vi "TUNA midbrain THINK.vi"(3 "error in":errorcluster, 4 "Forebrain Comd":T2, 5 "IR Sensors":T3(array[cluster]), 6 "Camera Data":T1(array[cluster])) -> (0 "error out":errorcluster, 1 "Behavior\nVelocity OUT":dbl, 2 "Behavior arrays":T4)   [LabVIEW 2014]
doc: "This vi is the midbrain THINK routine. It selects the behaviors which the boat will use based upon the passed Forebrain Command."
panel:
  out "Waveform Graph":cluster{dbl, dbl, dbl[][]}(graph)
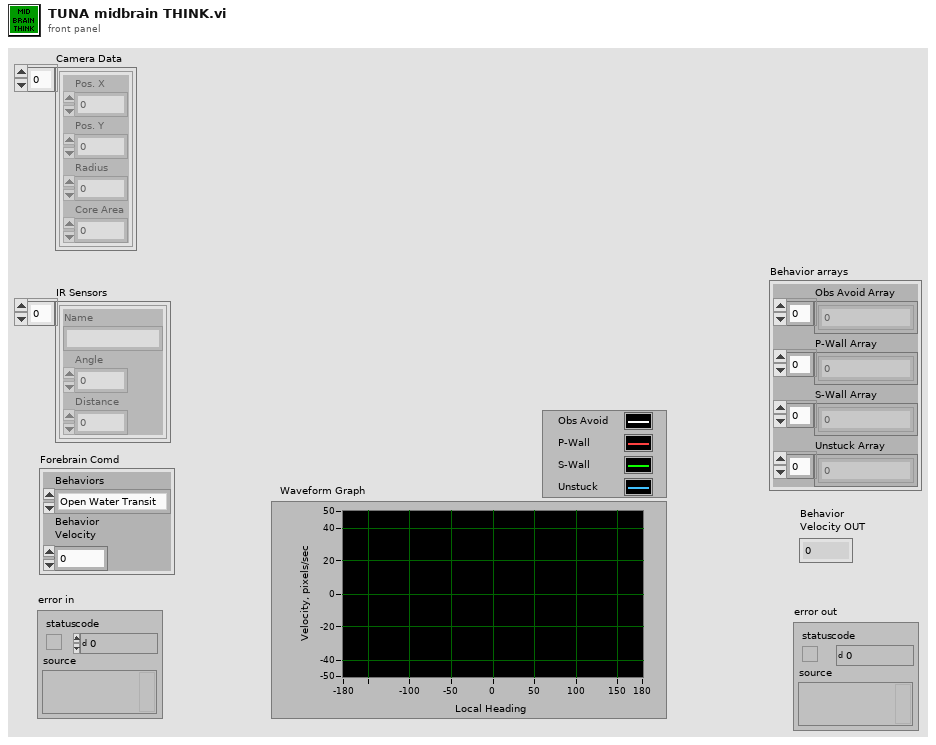
[diagram p1: front panel]
types:
  T1 = cluster{"Pos. X":i32, "Pos. Y":i32, "Radius":i32, "Core Area":i32}[]
  T2 = cluster{"Behaviors":enum16{"Open Water Transit", "P-Wall Follow", "S-Wall Follow", "Dock"}, "Behavior\nVelocity":dbl}
  T3 = cluster{"Name":string, "Angle":dbl, "Distance":dbl}[]
  T4 = cluster{"Obs Avoid Array":dbl[], "P-Wall Array":dbl[], "S-Wall Array":dbl[], "Unstuck Array":dbl[]}
  T5 = enum16{"Open Water Transit", "P-Wall Follow", "S-Wall Follow", "Dock"}
  T6 = cluster{"Obstacle Avoidance":bool, "P-Wall Follow":bool, "S-Wall Follow":bool, "Point to Dock":bool}
  T7 = cluster{"Obs Avoid Array":dbl[], "P-Wall Array":dbl[], "S-Wall Array":dbl[], "Dock Array":dbl[]}
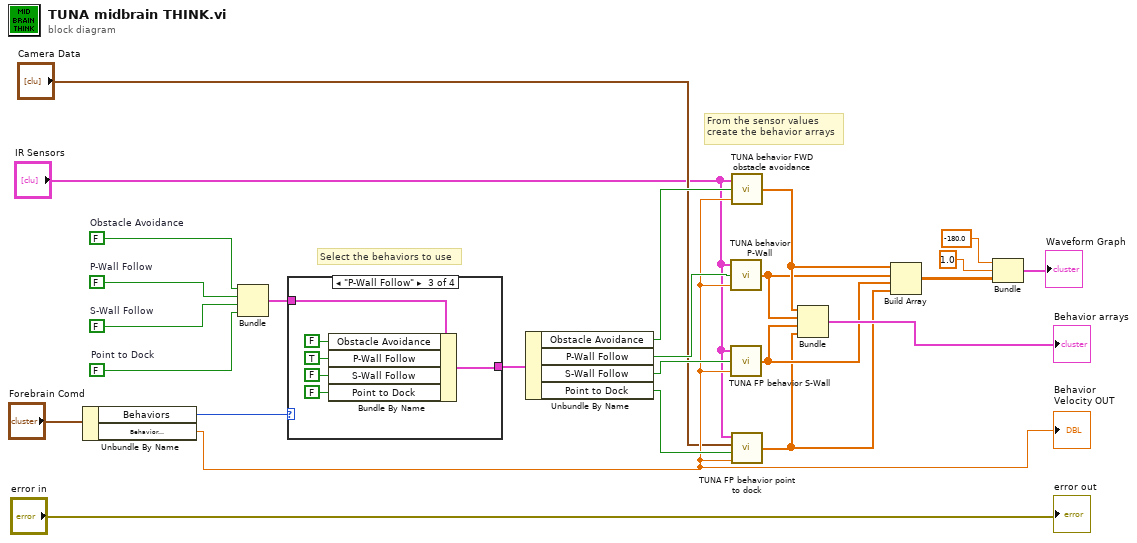
[diagram p0: block diagram]
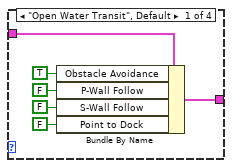
[diagram p2: hidden frame]
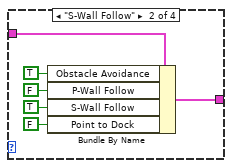
[diagram p3: hidden frame]
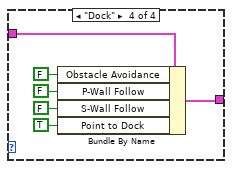
[diagram p4: hidden frame]
diagram:
  w21 = FALSE  # Point to Dock
  w22 = FALSE  # S-Wall Follow
  w23 = FALSE  # P-Wall Follow
  w24 = FALSE  # Obstacle Avoidance
  # "From the sensor values\ncreate the behavior arrays"
  # "Select the behaviors to use"
  n1 = Unbundle By Name("Forebrain Comd") -> ("Behaviors"=w4:T5, "Behavior\nVelocity"=w13:dbl)
  "Behavior\nVelocity OUT" <- w13
  n2 = Bundle("Obstacle Avoidance"=w24, "P-Wall Follow"=w23, "S-Wall Follow"=w22, "Point to Dock"=w21) -> (w20:T6)  [unwired: 1 in]
  n3 = case shown="\"P-Wall Follow\"" w4 {
    tunnel: w20 -> [w31 w37 w43 w49]
    tunnel: [w29 w35 w41 w47] -> w19
    frame "Open Water Transit", Default {
      n4 = Bundle By Name(cluster=w31, "Obstacle Avoidance"=TRUE, "P-Wall Follow"=FALSE, "S-Wall Follow"=FALSE, "Point to Dock"=FALSE ("Get Unstuck")) -> (w29:T6)
    }
    frame "S-Wall Follow" {
      n5 = Bundle By Name(cluster=w37, "Obstacle Avoidance"=TRUE, "P-Wall Follow"=FALSE, "S-Wall Follow"=TRUE, "Point to Dock"=FALSE ("Get Unstuck")) -> (w35:T6)
    }
    frame "P-Wall Follow" {
      n6 = Bundle By Name(cluster=w43, "Obstacle Avoidance"=FALSE, "P-Wall Follow"=TRUE, "S-Wall Follow"=FALSE, "Point to Dock"=FALSE ("Get Unstuck")) -> (w41:T6)
    }
    frame "Dock" {
      n7 = Bundle By Name(cluster=w49, "Obstacle Avoidance"=FALSE, "P-Wall Follow"=FALSE, "S-Wall Follow"=FALSE, "Point to Dock"=TRUE ("Get Unstuck")) -> (w47:T6)
    }
  }
  n8 = Unbundle By Name(w19) -> ("Obstacle Avoidance"=w18:bool, "P-Wall Follow"=w15:bool, "S-Wall Follow"=w16:bool, "Point to Dock"=w17:bool)
  n9 = call "TUNA behavior P-Wall.vi"("Behavior\nVelocity"=w13, "Activate?"=w15, "IR Sensors"="IR Sensors") -> ("P-Wall Array"=w8:dbl[])
  n10 = call "TUNA FP behavior S-Wall.vi"("Behavior\nVelocity"=w13, "Activate?"=w16, "IR Sensors"="IR Sensors") -> ("S-Wall Array"=w6:dbl[])
  n11 = call "TUNA behavior FWD obstacle avoidance.vi"("Behavior\nVelocity"=w13, "Activate?"=w18, "IR Sensors"="IR Sensors") -> ("Obs Avoid Array"=w9:dbl[])
  n12 = call "TUNA FP behavior point to dock.vi"("Behavior\nVelocity"=w13, "Activate?"=w17, "Camera Data"="Camera Data", "IR Sensors"="IR Sensors") -> ("Dock Array"=w5:dbl[])
  n13 = Bundle("Obs Avoid Array"=w9, "P-Wall Array"=w8, "S-Wall Array"=w6, "Dock Array"=w5) -> (→"Behavior arrays":T7)  [unwired: 1 in]
  n14 = Build Array(w9, w8, w6, w5) -> (w7:dbl[][])
  n15 = Bundle(-180.0, 1.0, w7) -> (→"Waveform Graph":cluster{dbl, dbl, dbl[][]})  [unwired: 1 in]
  "error out" <- "error in"
